vi "Save_Config.vi"   [LabVIEW 2016]
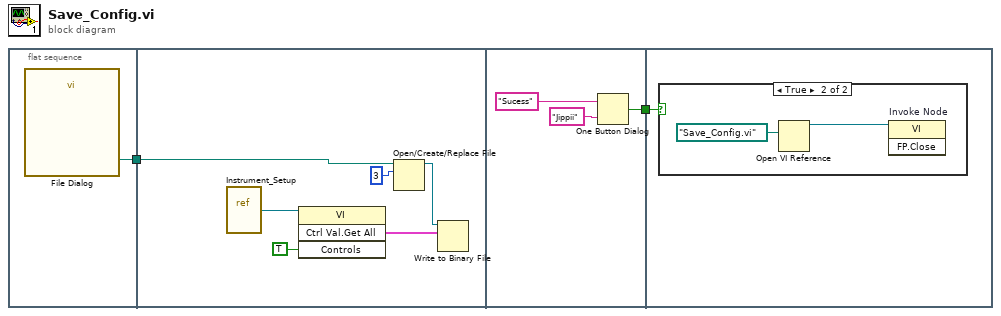
[diagram p0: block diagram]
diagram:
  n1 = flat-sequence {
    tunnel: [w3] -> w1
    tunnel: w1 -> [w4]
    tunnel: [w10] -> w2
    tunnel: w2 -> [w13]
    frame #0 {
      n2 = call "File Dialog"() -> ("selected path"=w3:path)  [unwired: 12 in, 3 out]
    }
    frame #1 {
      n3 = vi-ref "Instrument_Setup.vi"() -> (w8:refnum<vi>)
      n4 = invoke class="VI" method="Ctrl Val.Get All"(reference=w8, "Controls"=TRUE) -> ("Get All Control Values Variant"=w5:cluster{"Name":string, "Variant Data":variant}[])  [unwired: 2 in, 3 out]
      n5 = Open/Create/Replace File(file path (use dialog)=w4, operation (0:open)=3) -> (refnum out=w6:refnum<file>)  [unwired: 4 in, 2 out]
      n6 = Write to Binary File(file (use dialog)=w6, data=w5) -> ()  [unwired: 4 in, 3 out]
    }
    frame #2 {
      n7 = One Button Dialog(message="Sucess", button name ("OK")="Jippii") -> (true=w10:bool)
    }
    frame #3 {
      n8 = case shown="True" w13 {
        frame False {
        }
        frame True {
          n9 = Open VI Reference(vi path=path "Save_Config.vi") -> (vi reference=w14:refnum<vi>)  [unwired: 5 in, 1 out]
          n10 = invoke on="Invoke Node" class="VI" method="FP.Close"(reference=w14) -> ()  [unwired: 2 in, 3 out]
        }
      }
    }
  }
